vi "templateFSM.vi"() -> ()   [LabVIEW 2018]
uses:
  enumMsgTemplate.ctl
  enumFsmTemplate.ctl
  controls/enumFgvFunctionFsm.ctl
panel:
  in  "시스템 정지":bool
  out "Template 통신":bool
  out "Template 상태":string
  out "Template 루프시간":timestamp format="%<%H:%M:%S%3u>T"
  in  "Template 루프타이머(ms)":u32=10
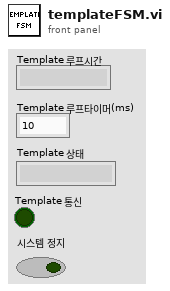
[diagram p1: front panel]
types:
  T1 = typedef "enumFgvFunctionFsm.ctl" = enum16{"Open", "Read", "Check", "Clear", "Write", "Close"}
  T2 = typedef "enumFsmTemplate.ctl" = enum16{"장치 열기", "장치 설정", "장치 읽기", "장치 쓰기", "장치 닫기", "대기", "에러"}
  T3 = typedef "enumMsgTemplate.ctl" = enum16{"", "접속중", "설정중", "통신에러", "종료", "통신중", "대기", "에러", "재접속중"}
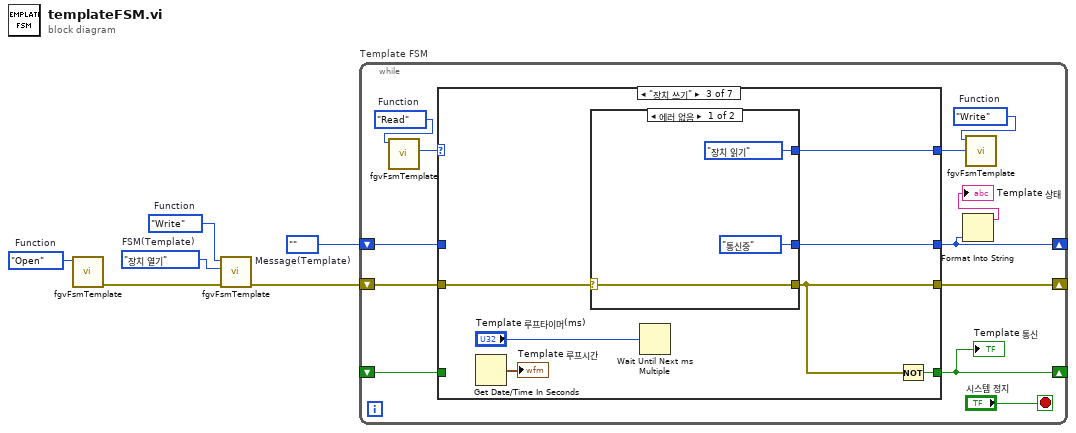
[diagram p0: block diagram]
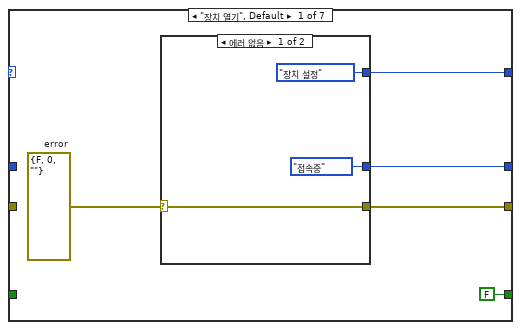
[diagram p2: hidden frame]
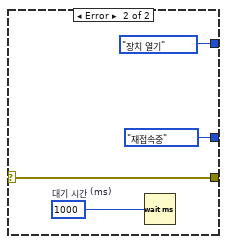
[diagram p3: hidden frame]
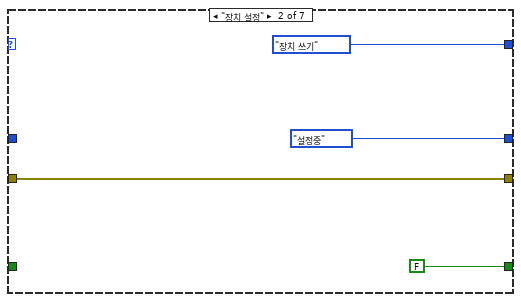
[diagram p4: hidden frame]
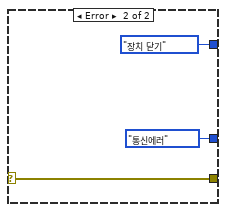
[diagram p5: hidden frame]
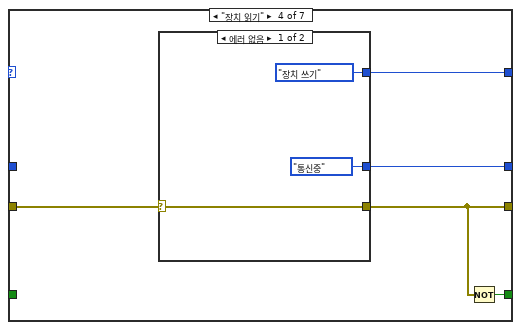
[diagram p6: hidden frame]
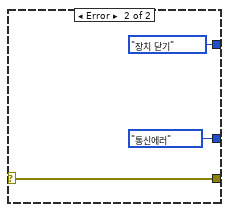
[diagram p7: hidden frame]
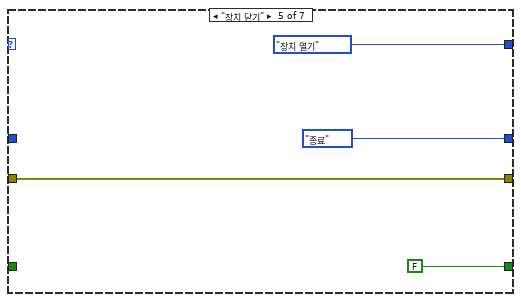
[diagram p8: hidden frame]
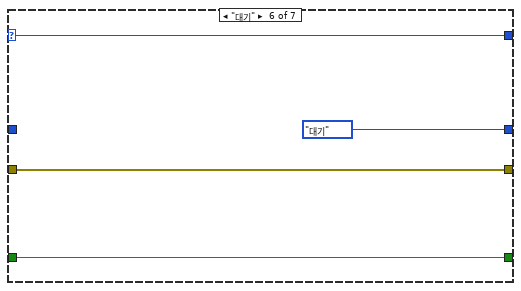
[diagram p9: hidden frame]
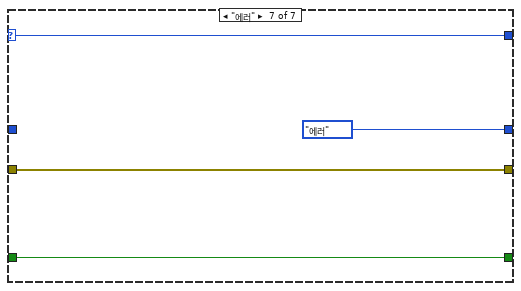
[diagram p10: hidden frame]
diagram:
  w2 = enumFgvFunctionFsm."Write"  # Function
  w4 = enumFgvFunctionFsm."Open"  # Function
  w5 = enumFsmTemplate."장치 열기"  # FSM(Template)
  w6 = enumMsgTemplate.""  # Message(Template)
  n1 = call "fgvFsmTemplate.vi"("Function"=w4) -> ("Error Out"=w3:errorcluster)  [unwired: 8 in, 2 out]
  n2 = call "fgvFsmTemplate.vi"("Error In"=w3, "Write"=w5, "Function"=w2) -> ("Error Out"=w1:errorcluster)  [unwired: 6 in, 2 out]
  n3 = while "Template FSM" {
    shift-right: [w18] -> _
    shift-left: w1 -> [w17]
    shift-right: [w14] -> _
    shift-left: w6 -> [w16]
    shift-right: [w12] -> _
    shift-left: _ -> [w15]
    stop <- "시스템 정지" stop-if-true
    w7 = enumFgvFunctionFsm."Write"  # Function
    w9 = enumFgvFunctionFsm."Read"  # Function
    n4 = call "fgvFsmTemplate.vi"("Function"=w9) -> ("Read"=w10:T2)  [unwired: 8 in, 2 out]
    n5 = case shown="\"장치 쓰기\"" w10 {
      selector: w10 -> [_ _ _ _ _ w65 w70]
      tunnel: [w23 w32 w37 w50 w59 w66 w69] -> w18
      tunnel: w17 -> [_ w32 w41 w51 w59 w66 w69]
      tunnel: [w22 enumFsmTemplate."장치 쓰기" ("FSM(Template)") w40 w49 enumFsmTemplate."장치 열기" ("FSM(Template)") w65 w70] -> w8
      tunnel: [w21 enumMsgTemplate."설정중" ("Message(Template)") w39 w48 enumMsgTemplate."종료" ("Message(Template)") enumMsgTemplate."대기" ("Message(Template)") enumMsgTemplate."에러" ("Message(Template)")] -> w14
      tunnel: w16 -> [_ _ _ _ _ _ _]
      tunnel: w15 -> [_ _ _ _ _ w64 w68]
      tunnel: [FALSE FALSE w38 w52 FALSE w64 w68] -> w12
      frame "장치 열기", Default {
        w20 = errorcluster {"status"=FALSE, "code"=0, "source"=""}  # error
        n6 = case shown="에러 없음" w20 {
          selector: w20 -> [w26 w30]
          tunnel: [w26 w30] -> w23
          tunnel: [enumFsmTemplate."장치 설정" ("FSM(Template)") enumFsmTemplate."장치 열기" ("FSM(Template)")] -> w22
          tunnel: [enumMsgTemplate."접속중" ("Message(Template)") enumMsgTemplate."재접속중" ("Message(Template)")] -> w21
          frame No Error {
          }
          frame Error {
            w29 = u32 1000  # 대기 시간 (ms)
            n7 = Wait (ms)(milliseconds to wait=w29) -> ()  [unwired: 1 out]
          }
        }
      }
      frame "장치 설정" {
      }
      frame "장치 쓰기" {
        n8 = Get Date/Time In Seconds() -> (seconds since 1Jan1904=→"Template 루프시간":timestamp)
        n9 = case shown="에러 없음" w41 {
          selector: w41 -> [w42 w46]
          tunnel: [w42 w46] -> w37
          tunnel: [enumFsmTemplate."장치 읽기" ("FSM(Template)") enumFsmTemplate."장치 닫기" ("FSM(Template)")] -> w40
          tunnel: [enumMsgTemplate."통신중" ("Message(Template)") enumMsgTemplate."통신에러" ("Message(Template)")] -> w39
          frame No Error {
          }
          frame Error {
          }
        }
        n10 = Wait Until Next ms Multiple(millisecond multiple="Template 루프타이머(ms)") -> ()  [unwired: 1 out]
        n11 = Not(x=w37) -> (.not. x?=w38:bool)
      }
      frame "장치 읽기" {
        n12 = case shown="에러 없음" w51 {
          selector: w51 -> [w55 w56]
          tunnel: [w55 w56] -> w50
          tunnel: [enumFsmTemplate."장치 쓰기" ("FSM(Template)") enumFsmTemplate."장치 닫기" ("FSM(Template)")] -> w49
          tunnel: [enumMsgTemplate."통신중" ("Message(Template)") enumMsgTemplate."통신에러" ("Message(Template)")] -> w48
          frame No Error {
          }
          frame Error {
          }
        }
        n13 = Not(x=w50) -> (.not. x?=w52:bool)
      }
      frame "장치 닫기" {
      }
      frame "대기" {
      }
      frame "에러" {
      }
    }
    "Template 통신" <- w12
    n14 = Format Into String(w14) -> (resulting string=→"Template 상태":string)  [unwired: 3 in, 1 out]
    n15 = call "fgvFsmTemplate.vi"("Write"=w8, "Function"=w7) -> ()  [unwired: 7 in, 3 out]
  }
